vi "I2C_ReadBlockData.vi"(5 "Bus":i32=1, 6 "Device register":u8 format="%.0x", 7 "Address":u8 format="%.0x", 8 "error in":errorcluster, 11 "length":i32=32) -> (0 "error out":errorcluster, 4 "Block":u16[](array[numeric]) format="%.0x")   [LabVIEW 2014, in "GPIO.lvlib"]
uses:
  GPIO.lvlib
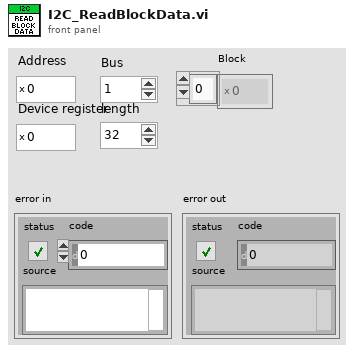
[diagram p1: front panel]
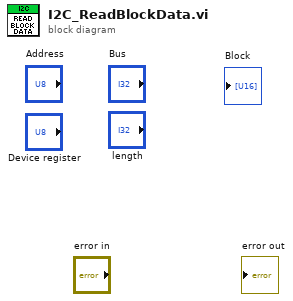
[diagram p0: block diagram]
diagram:
